vi "TestSubvi.vi"() -> (3 "Waveform Chart":dbl(graph))   [LabVIEW 2023]
panel:
  in  "Stop Button":bool
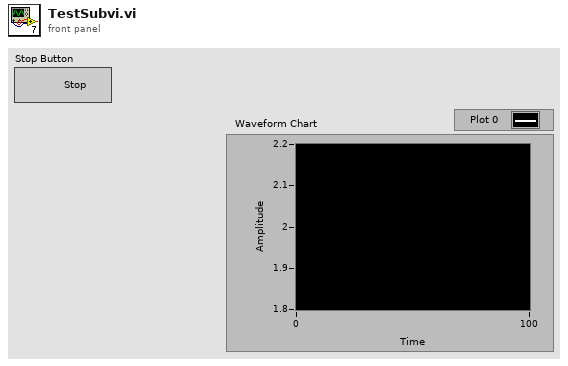
[diagram p1: front panel]
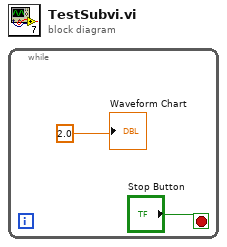
[diagram p0: block diagram]
diagram:
  n1 = while {
    stop <- "Stop Button" stop-if-true
    "Waveform Chart" <- 2.0 ("Waveform Chart")
  }
